vi "Shut Down Async Loops.vi"(0 "VI Refs":refnum<vi>[](array[refnum])) -> ()   [LabVIEW 2016, in "Ballard Arinc-429 Engine.lvlib"]
uses:
  Ballard Arinc-429 Engine.lvlib
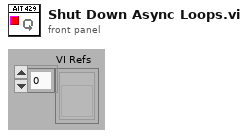
[diagram p1: front panel]
types:
  T1 = enum32{"Bad", "Idle", "Run top level", "Running"}
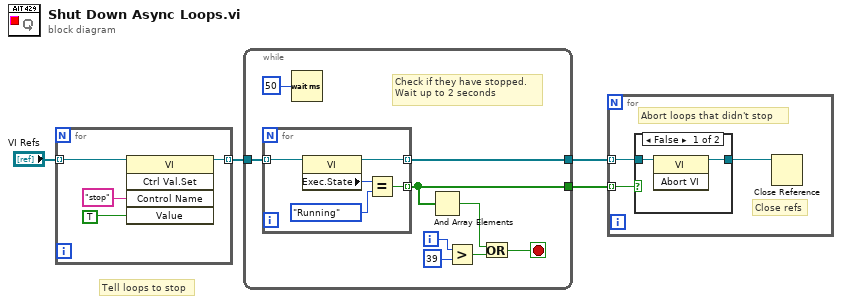
[diagram p0: block diagram]
diagram:
  # "Tell loops to stop"
  n1 = for {
    tunnel: "VI Refs" -> [w8] mode=indexing
    tunnel: [w6] -> w3 mode=indexing
    n2 = invoke class="VI" method="Ctrl Val.Set"(reference=w8, "Control Name"="stop", "Value"=TRUE ("force destroy? (F)")) -> (reference out=w6:refnum<vi>)  [unwired: 2 in, 4 out]
  }
  n3 = while {
    tunnel: w3 -> [w16]
    tunnel: [w15] -> w1
    tunnel: [w10] -> w2
    i -> [w13]
    stop <- w14 stop-if-true
    # "Check if they have stopped.\nWait up to 2 seconds"
    n4 = for {
      tunnel: w16 -> [w22] mode=indexing
      tunnel: [w18] -> w10 mode=indexing
      tunnel: [w21] -> w15 mode=indexing
      n5 = property class="VI"(reference=w22) -> (reference out=w21:refnum<vi>, "Exec.State"=w20:T1)  [unwired: 1 in, 1 out]
      n6 = Equal?(x=w20, y=T1."Running") -> (x = y?=w18:bool)
    }
    n7 = Wait (ms)(milliseconds to wait=u32 50) -> ()  [unwired: 1 out]
    n8 = And Array Elements(Boolean array=w10) -> (logical AND=w9:bool)
    n9 = Greater?(x=w13, y=39) -> (0:w11:bool)
    n10 = Or(x=w9, y=w11) -> (x .or. y?=w14:bool)
  }
  n11 = for {
    tunnel: w1 -> [w25] mode=indexing
    tunnel: w2 -> [w24] mode=indexing
    # "Close refs"
    # "Abort loops that didn't stop"
    n12 = case shown="False" w24 {
      tunnel: w25 -> [w27 w28]
      tunnel: [w26 w28] -> w23
      frame False {
        n13 = invoke class="VI" method="Abort VI"(reference=w27) -> (reference out=w26:refnum<vi>)  [unwired: 2 in, 2 out]
      }
      frame True {
      }
    }
    n14 = Close Reference(reference=w23) -> ()  [unwired: 1 in, 1 out]
  }
